vi "Initalize.vi"(8 "error in (no error)":errorcluster, 9 "Section":string, 10 "Config Path":path, 11 "SIM Motion Controller in":refnum<class "Fine SIM Motion Controller.lvclass">) -> (0 "error out":errorcluster, 3 "SIM Motion Controller out":refnum<class "Fine SIM Motion Controller.lvclass">)   [LabVIEW 2022 SP3, in "Fine SIM Motion Controller.lvclass"]
uses:
  Fine SIM Motion Controller.lvclass
  Motion Controller/Parent SIM Motion Controller.lvclass
  Fine SIM Motion Controller.lvclass/Fine SIM Motion Controller.ctl
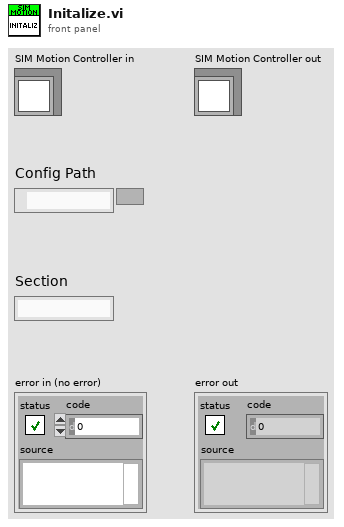
[diagram p1: front panel]
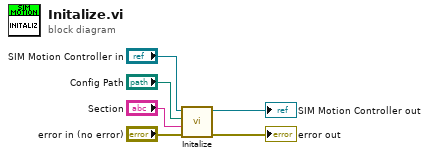
[diagram p0: block diagram]
diagram:
  n1 = call-parent "Initalize.vi"("error in (no error)"="error in (no error)", "Section"="Section", "Config Path"="Config Path", "Motion Controller in"="SIM Motion Controller in") -> ("error out"=→"error out":errorcluster, "Motion Controller out"=→"SIM Motion Controller out":refnum<class "Fine SIM Motion Controller.lvclass">)  [unwired: 6 in]
